vi "报警信息数据插入.vi"(0 "data":T1, 3 "错误输入（无错误）":errorcluster) -> (10 "错误输出":errorcluster)   [LabVIEW 2016]
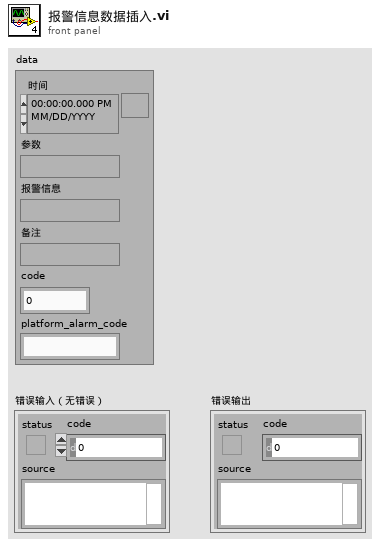
[diagram p1: front panel]
types:
  T1 = typedef "报警信息字段定义.ctl" = cluster{"时间":timestamp, "参数":string, "报警信息":string, "备注":string, "code":u64, "platform_alarm_code":string}
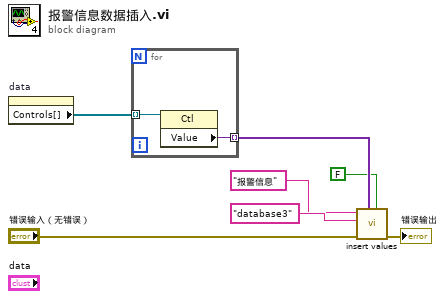
[diagram p0: block diagram]
diagram:
  n1 = property on="data" class="Clust (严格)"() -> ("Controls[]"=w7:refnum<vi>[])  [unwired: 2 in, 2 out]
  n2 = for {
    tunnel: w7 -> [w9] mode=indexing
    tunnel: [w8] -> w6 mode=indexing
    n3 = property class="Ctl"(reference=w9) -> ("Value"=w8:variant)  [unwired: 1 in, 2 out]
  }
  n4 = call "insert values.vi"("是否创建唯一键"=FALSE, "data"=w6, "错误输入（无错误）"="错误输入（无错误）", "database"="database3", "Tabe Name"="报警信息") -> ("错误输出"=→"错误输出":errorcluster)  [unwired: 6 in]
